vi "ESP8266 UDP Server Writing Samples As Bytes.vi"() -> ()   [LabVIEW 2014]
uses:
  <vilib>/LabVIEW Universal Transcriptor/LabVIEW to Arduino Transcriptor/Transcriptors/System API/Serial println string.vi
  <vilib>/LabVIEW Universal Transcriptor/ESP8266 WiFi Wrapper/ESP8266 WiFi Wrapper.lvlib
  <vilib>/LabVIEW Universal Transcriptor/Arduino MPU6050 Library/Arduino MPU6050.lvlib
panel:
  out "Chars written":u8
  out "Error Out":errorcluster
  in  "DNS address":u8[](array[numeric])=[0, 0, 0, 0]
  in  "IP address":u8[](array[numeric])=[192, 168, 0, 47]
  in  "Gateway":u8[](array[numeric])=[192, 168, 0, 1]
  in  "Subnet mask":u8[](array[numeric])=[255, 255, 255, 0]
  in  "Password":string="12345678"
  in  "SSID":string="ESP8266 Wifi UDP"
  in  "Listen Port":i16=8080
  in  "error in (no error)":errorcluster
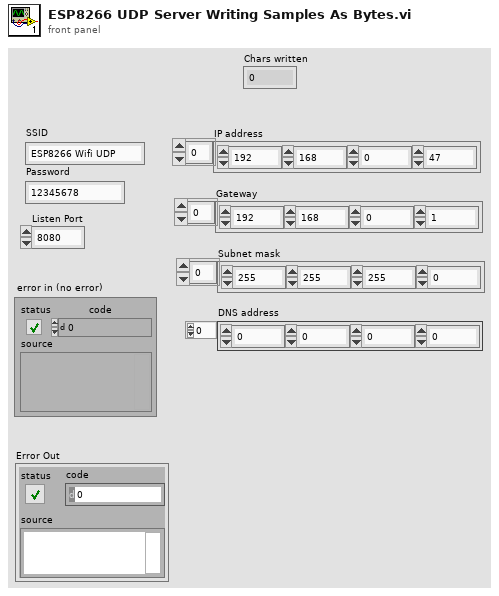
[diagram p1: front panel]
types:
  T1 = enum16{"MPU6050_SCALE_250DPS", "MPU6050_SCALE_500DPS", "MPU6050_SCALE_1000DPS", "MPU6050_SCALE_2000DPS"}
  T2 = enum16{"MPU6050_RANGE_2G", "MPU6050_RANGE_4G", "MPU6050_RANGE_8G", "MPU6050_RANGE_16G"}
  T3 = enum16{"WIFI_OFF", "WIFI_STA", "WIFI_AP", "WIFI_AP_STA"}
  T4 = typedef "Arduino MPU6050.lvlib/MPU6050LibVector.ctl" = cluster{"XAxis":sgl, "YAxis":sgl, "ZAxis":sgl}
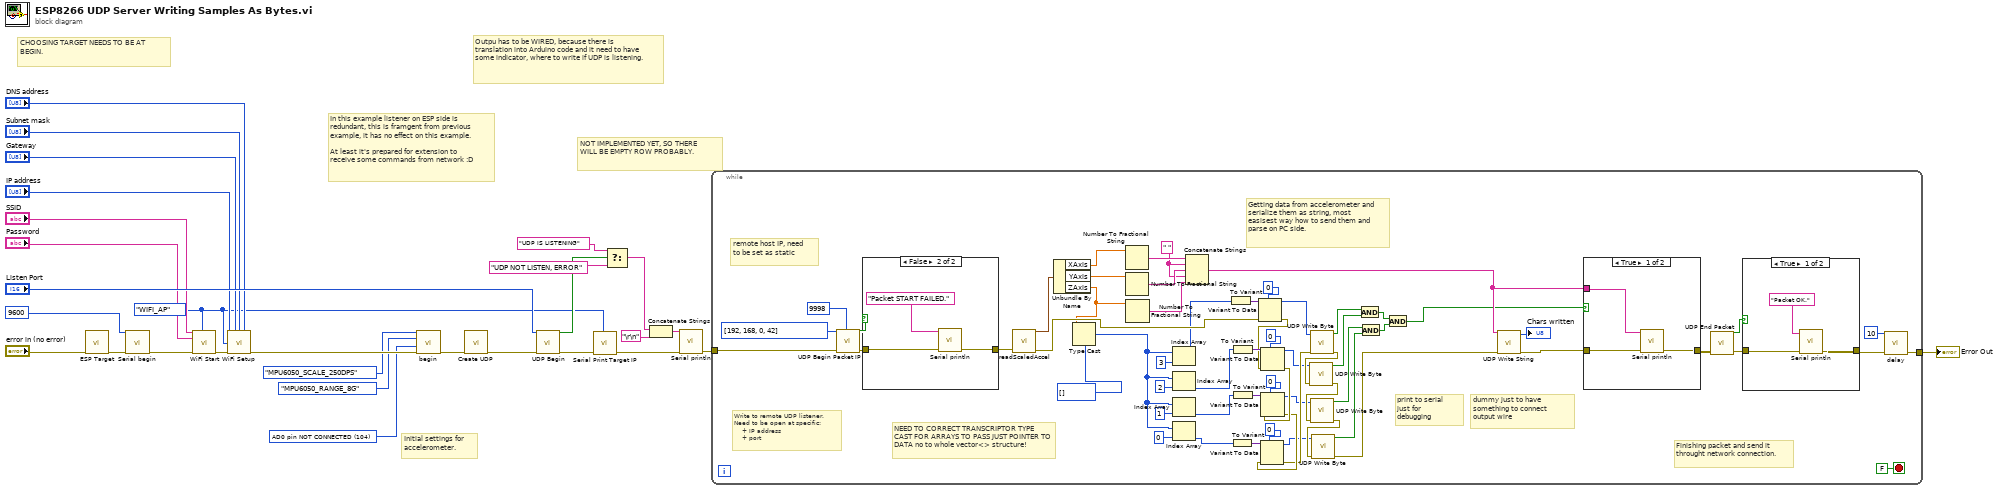
[diagram p0: block diagram]
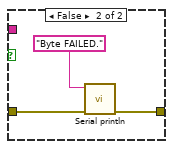
[diagram p2: hidden frame]
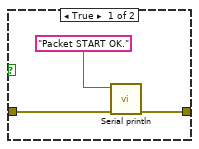
[diagram p3: hidden frame]
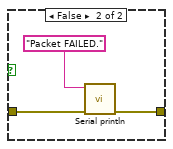
[diagram p4: hidden frame]
diagram:
  w3 = u16 104 items=["AD0 pin NOT CONNECTED"=104, "AD0 connect to Vcc"=105] ("address")
  w6 = T3."WIFI_AP" ("WiFi Mode")
  # "In this example listener on ESP side is redundant, this is framgent from previous example, it has no effect on this example.\n\nAt least it's prepared for extension to receive some commands from network :D"
  # "Initial settings for accelerometer."
  # "NOT IMPLEMENTED YET, SO THERE WILL BE EMPTY ROW PROBABLY."
  # "Outpu has to be WIRED, because there is translation into Arduino code and it need to have some indicator, where to write if UDP is listening."
  # "CHOOSING TARGET NEEDS TO BE AT BEGIN."
  n1 = call <vilib>:"ESP Target.vi"("Error In"="error in (no error)") -> ("Error Out"=w28:errorcluster)  [unwired: 10 in]
  n2 = call <vilib>:"Serial begin.vi"("Error In"=w28, "speed (Bd)"=u32 9600 ("Speed")) -> ("Error Out"=w19:errorcluster)  [unwired: 9 in]
  n3 = call <vilib>:"WiFi Start.vi"("WiFi Mode"=w6, "Error In"=w19, "Password"="Password", "SSID"="SSID") -> ("Error Out"=w18:errorcluster)  [unwired: 7 in]
  n4 = call <vilib>:"WiFi Setup.vi"("IP address"="IP address", "Gateway address"="Gateway", "Subnet mask"="Subnet mask", "DNS address"="DNS address", "WiFi Mode"=w6, "Error In"=w18) -> ("Error Out"=w5:errorcluster)  [unwired: 9 in]
  n5 = call <vilib>:"begin.vi"("Error In"=w5, "address"=w3, "range"=T2."MPU6050_RANGE_8G", "scale"=T1."MPU6050_SCALE_250DPS") -> ("Error Out"=w4:errorcluster)  [unwired: 7 in]
  n6 = call <vilib>:"Create UDP.vi"("Error In"=w4) -> ("Error Out"=w17:errorcluster)  [unwired: 10 in]
  n7 = call <vilib>:"UDP Begin.vi"("Error In"=w17, "Port"="Listen Port") -> ("Error Out"=w8:errorcluster, "Is listening?"=w13:bool)  [unwired: 8 in]
  n8 = call <vilib>:"Serial Print Target IP.vi"("WiFi Mode"=w6, "Error In"=w8) -> ("Error Out"=w7:errorcluster)  [unwired: 9 in]
  n9 = Select(t="UDP IS LISTENING", s=w13, f="UDP NOT LISTEN, ERROR") -> (s? t:f=w10:string)
  n10 = Concatenate Strings(w10, "\r\n") -> (w12:string)
  n11 = call-poly <vilib>:"Serial println.vi"("Error In"=w7, "string in"=w12) -> ("Error Out"=w16:errorcluster)  [unwired: 9 in]
  n12 = while {
    tunnel: w16 -> [w88]
    tunnel: [w89] -> w9
    stop <- FALSE stop-if-true
    w71 = " " ("string")
    # "NEED TO CORRECT TRANSCRIPTOR TYPE CAST FOR ARRAYS TO PASS JUST POINTER TO DATA no to whole vector<> structure!"
    # "dummy just to have something to connect output wire"
    # "print to serial just for debugging"
    # "remote host IP, need to be set as static"
    # "Finishing packet and send it throught network connection."
    # "Getting data from accelerometer and serialize them as string, most easisest way how to send them and parse on PC side."
    # "Write to remote UDP listener.\nNeed to be open at specific:\n    + IP address\n    + port"
    n13 = call <vilib>:"UDP Begin Packet IP.vi"("Port"=i16 9998, "Error In"=w88, "IP Address"=u8[] [192, 168, 0, 42]) -> ("Error Out"=w82:errorcluster, "Successful?"=w81:bool)  [unwired: 7 in]
    n14 = case shown="False" w81 {
      tunnel: w82 -> [w100 w103]
      tunnel: [w99 w102] -> w79
      frame True {
        n15 = call-poly <vilib>:"Serial println.vi"("Error In"=w100, "string in"="Packet START OK.") -> ("Error Out"=w99:errorcluster)  [unwired: 9 in]
      }
      frame False {
        n16 = call-poly <vilib>:"Serial println.vi"("Error In"=w103, "string in"="Packet START FAILED.") -> ("Error Out"=w102:errorcluster)  [unwired: 9 in]
      }
    }
    n17 = call <vilib>:"readScaledAccel.vi"("error in (no error)"=w79) -> ("error out"=w69:errorcluster, "Vector"=w78:T4)  [unwired: 9 in]
    n18 = Unbundle By Name(w78) -> ("XAxis"=w74:sgl, "YAxis"=w73:sgl, "ZAxis"=w32:sgl)
    n19 = Type Cast(type=u8[] [], x=w32) -> (*(type *) &x=w31:u8[])
    n20 = Number To Fractional String(number=w74) -> (F-format string=w77:string)  [unwired: 3 in]
    n21 = Number To Fractional String(number=w73) -> (F-format string=w76:string)  [unwired: 3 in]
    n22 = Number To Fractional String(number=w32) -> (F-format string=w75:string)  [unwired: 3 in]
    n23 = Index Array(array=w31, index=3) -> (element=w40:u8)
    n24 = Index Array(array=w31, index=2) -> (element=w39:u8)
    n25 = Index Array(array=w31, index=1) -> (element=w38:u8)
    n26 = Index Array(array=w31, index=0) -> (element=w37:u8)
    n27 = Concatenate Strings(w77, w71, w76, w71, w75) -> (w70:string)
    n28 = To Variant(anything=w40) -> (Variant=w45:variant)
    n29 = To Variant(anything=w37) -> (Variant=w48:variant)
    n30 = To Variant(anything=w39) -> (Variant=w52:variant)
    n31 = To Variant(anything=w38) -> (Variant=w49:variant)
    n32 = Variant To Data(error in=w69, type=u8 0 ("index"), Variant=w45) -> (data=w36:u8, error out=w44:errorcluster)
    n33 = Variant To Data(error in=w44, type=u8 0 ("index"), Variant=w52) -> (data=w35:u8, error out=w43:errorcluster)
    n34 = Variant To Data(error in=w43, type=u8 0 ("index"), Variant=w49) -> (data=w34:u8, error out=w42:errorcluster)
    n35 = Variant To Data(error in=w42, type=u8 0 ("index"), Variant=w48) -> (data=w33:u8, error out=w41:errorcluster)
    n36 = call <vilib>:"UDP Write Byte.vi"("Error In"=w41, "Byte to write"=w36) -> ("Error Out"=w68:errorcluster, "Byte written?"=w58:bool)  [unwired: 8 in]
    n37 = call <vilib>:"UDP Write Byte.vi"("Error In"=w68, "Byte to write"=w35) -> ("Error Out"=w67:errorcluster, "Byte written?"=w57:bool)  [unwired: 8 in]
    n38 = call <vilib>:"UDP Write Byte.vi"("Error In"=w67, "Byte to write"=w34) -> ("Error Out"=w66:errorcluster, "Byte written?"=w56:bool)  [unwired: 8 in]
    n39 = call <vilib>:"UDP Write Byte.vi"("Error In"=w66, "Byte to write"=w33) -> ("Error Out"=w65:errorcluster, "Byte written?"=w55:bool)  [unwired: 8 in]
    n40 = And(x=w58, y=w57) -> (x .and. y?=w59:bool)
    n41 = And(x=w56, y=w55) -> (x .and. y?=w60:bool)
    n42 = And(x=w59, y=w60) -> (x .and. y?=w53:bool)
    n43 = call <vilib>:"UDP Write String.vi"("Error In"=w65, "String to write"=w70) -> ("Error Out"=w72:errorcluster, "Chars written"=→"Chars written":u8)  [unwired: 8 in]
    n44 = case shown="True" w53 {
      tunnel: [w94 w97] -> w80
      tunnel: w72 -> [w92 w95]
      tunnel: w70 -> [w93 _]
      frame True {
        n45 = call-poly <vilib>:"Serial println.vi"("Error In"=w92, "string in"=w93) -> ("Error Out"=w94:errorcluster)  [unwired: 9 in]
      }
      frame False {
        n46 = call-poly <vilib>:"Serial println.vi"("Error In"=w95, "string in"="Byte FAILED.") -> ("Error Out"=w97:errorcluster)  [unwired: 9 in]
      }
    }
    n47 = call <vilib>:"UDP End Packet.vi"("Error In"=w80) -> ("Error Out"=w86:errorcluster, "Successful?"=w84:bool)  [unwired: 9 in]
    n48 = case shown="True" w84 {
      tunnel: w86 -> [w106 w109]
      tunnel: [w105 w108] -> w85
      frame True {
        n49 = call-poly <vilib>:"Serial println.vi"("Error In"=w106, "string in"="Packet OK.") -> ("Error Out"=w105:errorcluster)  [unwired: 9 in]
      }
      frame False {
        n50 = call-poly <vilib>:"Serial println.vi"("Error In"=w109, "string in"="Packet FAILED.") -> ("Error Out"=w108:errorcluster)  [unwired: 9 in]
      }
    }
    n51 = call <vilib>:"delay.vi"("Error In"=w85, "time (ms)"=10) -> ("Error Out"=w89:errorcluster)  [unwired: 9 in]
  }
  "Error Out" <- w9
